vi "New Server Socket from Context.vi"(8 "error in (no error)":errorcluster, 10 "TCP Refnum":refnum<k5>, 11 "SSL Server Ctx":refnum<class "SSL Server Context.lvclass">) -> (0 "error out":errorcluster, 3 "SSL Server Skt out":refnum<class "SSL Server Socket.lvclass">)   [LabVIEW 2013, in "OpenSSL Socket.lvlib" / "SSL Server Socket.lvclass"]
uses:
  SSL Server Socket.lvclass
  SSL Server Context/SSL Server Context.lvclass
  SSL_Lib/SSL/SSL_Mode.ctl
  SSL Context/SSL Context.lvclass/SSL Context.ctl
  Secure Socket/SSL Socket.lvclass/SSL Socket.ctl
  SSL Context/Read SSL Context.vi
  Secure Socket/Write BIO.vi
  SSL_Lib/SSL-Context/SSL-Context.lvclass
  SSL_Lib/SSL/SSL.lvclass
  SSL_Lib/BIO/BIO.lvclass
  SSL_Lib/SSL-Lib/SSL-Lib.lvclass
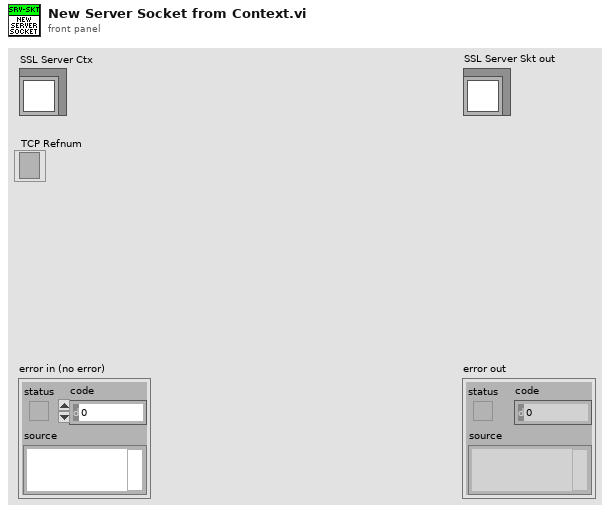
[diagram p1: front panel]
types:
  T1 = typedef "SSL_Lib.lvlib/SSL.lvclass/SSL_Mode.ctl" = i32
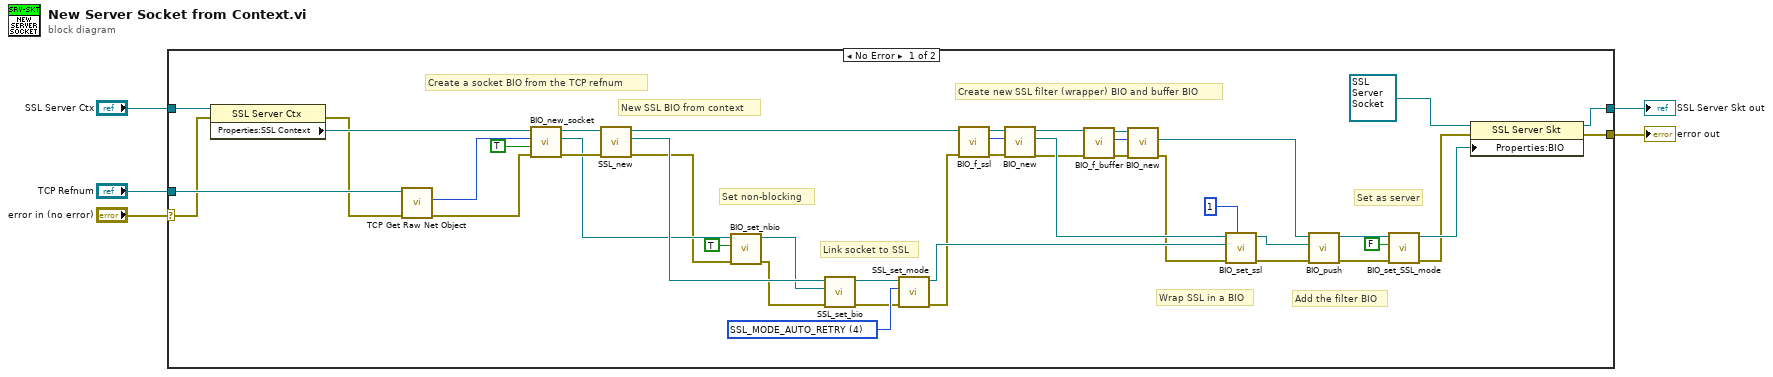
[diagram p0: block diagram]
diagram:
  n1 = case shown="No Error" "error in (no error)" {
    selector: "error in (no error)" -> [w20 w50]
    tunnel: [w6 w50] -> w4
    tunnel: [w8 _] -> w3
    tunnel: "SSL Server Ctx" -> [w23 _]
    tunnel: "TCP Refnum" -> [w49 _]
    frame No Error {
      w48 = T1 4 items=["None"=0, "SSL_MODE_ENABLE_PARTIAL_WRITE"=1, "SSL_MODE_ACCEPT_MOVING_WRITE_BUFFER"=2, "SSL_MODE_AUTO_RETRY"=4, "SSL_MODE_RELEASE_BUFFERS"=16, "SSL_MODE_SEND_FALLBACK_SCSV"=128] ("Mode")
      # "Set as server"
      # "Add the filter BIO"
      # "Wrap SSL in a BIO"
      # "Create new SSL filter (wrapper) BIO and buffer BIO"
      # "Link socket to SSL"
      # "Set non-blocking"
      # "New SSL BIO from context"
      # "Create a socket BIO from the TCP refnum"
      n2 = property class="SSL Server Ctx"(reference=w23, error in=w20) -> (error out=w19:errorcluster, "Properties:SSL Context"=w22:refnum<class "SSL-Context.lvclass">)  [unwired: 1 out]
      n3 = call <vilib>:"TCP Get Raw Net Object.vi"("error in (no error)"=w19, "connection ID"=w49) -> ("error out"=w18:errorcluster, "raw net object"=w21:u64)  [unwired: 7 in, 1 out]
      n4 = call "BIO_new_socket.vi"("error in (no error)"=w18, "Close on free? (T)"=TRUE, "fd"=w21, "SSL-Context in"=w22) -> ("error out"=w45:errorcluster, "Socket BIO out"=w42:refnum<class "BIO.lvclass">, "SSL-Context out"=w44:refnum<class "SSL-Context.lvclass">)  [unwired: 5 in]
      n5 = call "SSL_new.vi"("error in (no error)"=w45, "SSL-Context in"=w44) -> ("error out"=w39:errorcluster, "SSL out"=w43:refnum<class "SSL.lvclass">, "SSL-Context out"=w15:refnum<class "SSL-Context.lvclass">)  [unwired: 7 in]
      n6 = call "BIO_set_nbio.vi"("error in (no error)"=w39, "Non-Blocking?"=TRUE, "BIO in"=w42) -> ("error out"=w38:errorcluster, "BIO out"=w40:refnum<class "BIO.lvclass">)  [unwired: 7 in]
      n7 = call "SSL_set_bio.vi"("error in (no error)"=w38, "BIO"=w40, "SSL in"=w43) -> ("error out"=w37:errorcluster, "SSL out"=w41:refnum<class "SSL.lvclass">)  [unwired: 7 in]
      n8 = call "SSL_set_mode.vi"("error in (no error)"=w37, "Mode"=w48, "SSL in"=w41) -> ("error out"=w13:errorcluster, "SSL out"=w14:refnum<class "SSL.lvclass">)  [unwired: 7 in]
      n9 = call "BIO_f_ssl.vi"("error in (no error)"=w13, "SSL-Lib in"=w15) -> ("error out"=w33:errorcluster, "*BIO_Method"=w31:u64, "SSL-Lib out"=w32:refnum<class "SSL-Context.lvclass">)  [unwired: 7 in]
      n10 = call "BIO_new.vi"("error in (no error)"=w33, "*BIO_method"=w31, "SSL-Lib in"=w32) -> ("error out"=w16:errorcluster, "BIO out"=w30:refnum<class "BIO.lvclass">, "SSL-Lib out"=w12:refnum<class "SSL-Context.lvclass">)  [unwired: 6 in]
      n11 = call "BIO_f_buffer.vi"("error in (no error)"=w16, "SSL-Lib in"=w12) -> ("error out"=w36:errorcluster, "*BIO_Method"=w34:u64, "SSL-Lib out"=w35:refnum<class "SSL-Context.lvclass">)  [unwired: 7 in]
      n12 = call "BIO_new.vi"("error in (no error)"=w36, "*BIO_method"=w34, "SSL-Lib in"=w35) -> ("error out"=w11:errorcluster, "BIO out"=w28:refnum<class "BIO.lvclass">)  [unwired: 6 in, 1 out]
      n13 = call "BIO_set_ssl.vi"("close flag"=1, "error in (no error)"=w11, "SSL in"=w14, "BIO in"=w30) -> ("error out"=w17:errorcluster, "BIO out"=w27:refnum<class "BIO.lvclass">)  [unwired: 6 in]
      n14 = call "BIO_push.vi"("error in (no error)"=w17, "New BIO"=w27, "BIO in"=w28) -> ("error out"=w26:errorcluster, "BIO out"=w25:refnum<class "BIO.lvclass">)  [unwired: 7 in]
      n15 = call "BIO_set_SSL_mode.vi"("error in (no error)"=w26, "Client?"=FALSE, "BIO in"=w25) -> ("error out"=w7:errorcluster, "BIO out"=w9:refnum<class "BIO.lvclass">)  [unwired: 7 in]
      n16 = property class="SSL Server Skt"(reference=refnum<class "SSL Server Socket.lvclass"> refnum ("OpenSSL Socket.lvlib:SSL Server Skt"), error in=w7, "Properties:BIO"=w9) -> (reference out=w8:refnum<class "SSL Server Socket.lvclass">, error out=w6:errorcluster)
    }
    frame Error {
    }
  }
  "error out" <- w4
  "SSL Server Skt out" <- w3
